vi "plot_id_extractor.vi"(10 "Plot processed data In":T1={"Plot Rep Arrays"=[], "Graph Range Min/Max"={"X"={"Min"=0.0, "Max"=-inf}, "Y"={"Min"=0.0, "Max"=-inf}, "Z"={"Min"=inf, "Max"=-inf}, "Amplitude"={"Min"=0.0, "Max"=0.0}}} caption="Data In") -> (1 "Plot IDs":i32[](array[numeric]), 2 "Plot processed data Out":T1={"Plot Rep Arrays"=[], "Graph Range Min/Max"={"X"={"Min"=0.0, "Max"=-inf}, "Y"={"Min"=0.0, "Max"=-inf}, "Z"={"Min"=inf, "Max"=-inf}, "Amplitude"={"Min"=0.0, "Max"=0.0}}} caption="Data Out")   [LabVIEW 2020, in "3DPC_SurfacePlot.xctl"]
uses:
  <vilib>/Native 3D Graph/xcontrol/3DPC_SurfacePlot.xctl
  <vilib>/Native 3D Graph/xcontrol/Processed Data.ctl
  <vilib>/Native 3D Graph/typedefs/plot_rep_array.ctl
  <vilib>/Native 3D Graph/typedefs/plot_rep.ctl
  <vilib>/Native 3D Graph/typedefs/range_cluster.ctl
  <vilib>/Native 3D Graph/typedefs/min_max.ctl
  <vilib>/Native 3D Graph/typedefs/plot_rep_mesh_data.ctl
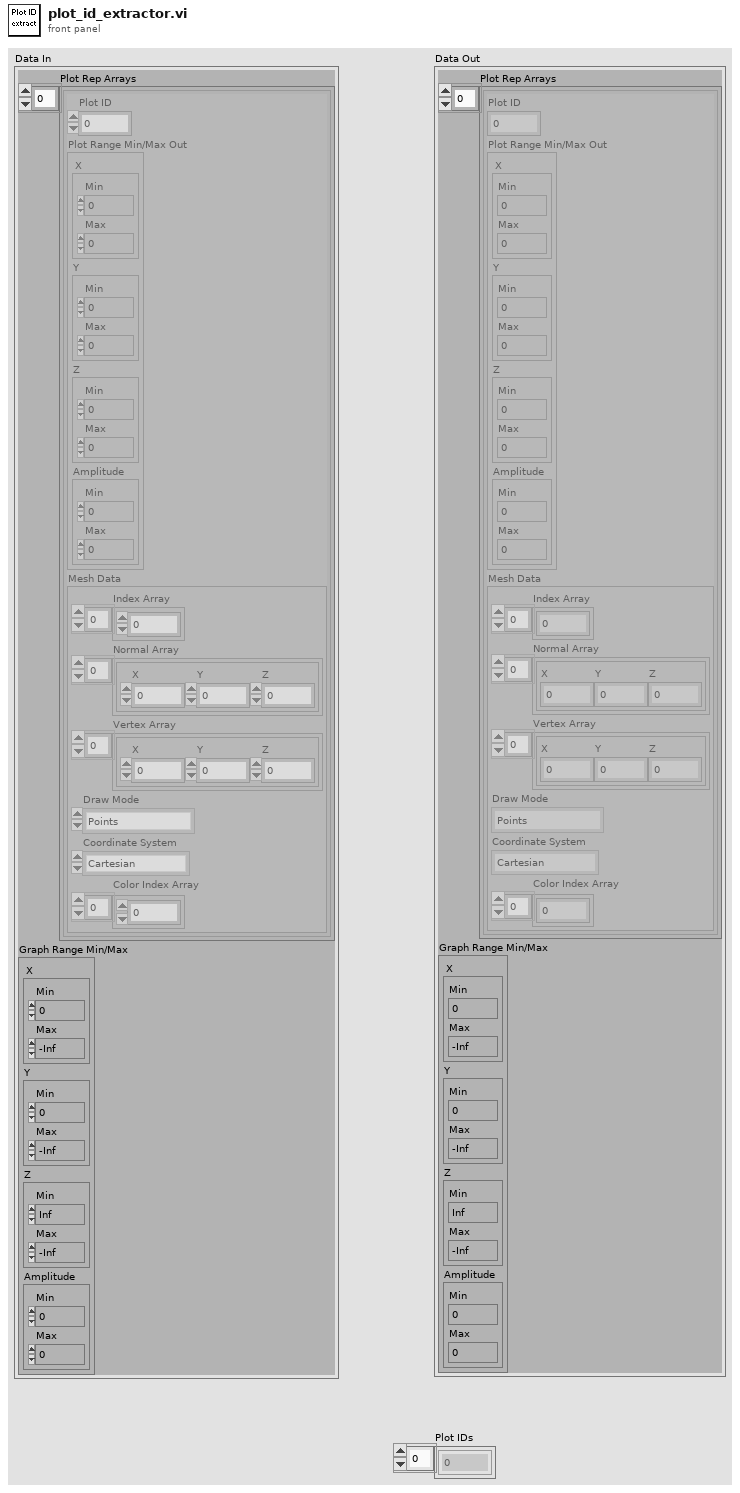
[diagram p1: front panel]
types:
  T1 = typedef "Processed Data.ctl" = cluster{"Plot Rep Arrays":T2, "Graph Range Min/Max":T4}
  T2 = typedef "3DPC_SurfacePlot.xctl/plot_rep_array.ctl" = T3[]
  T3 = typedef "3DPC_SurfacePlot.xctl/plot_rep.ctl" = cluster{"Plot ID":i32, "Plot Range Min/Max Out":T4, "Mesh Data":T6}
  T4 = typedef "3DPC_SurfacePlot.xctl/range_cluster.ctl" = cluster{"X":T5, "Y":T5, "Z":T5, "Amplitude":T5}
  T5 = typedef "3DPC_SurfacePlot.xctl/min_max.ctl" = cluster{"Min":sgl, "Max":sgl}
  T6 = typedef "3DPC_SurfacePlot.xctl/plot_rep_mesh_data.ctl" = cluster{"Index Array":u32[], "Normal Array":cluster{"X":sgl, "Y":sgl, "Z":sgl}[], "Vertex Array":cluster{"X":sgl, "Y":sgl, "Z":sgl}[], "Draw Mode":enum16{"Points", "Lines", "Line Strip", "Line Loop", "Triangles", "Triangle Strip", "Triangle Fan", "Quads", "Quad Strip", "Polygon"}, "Coordinate System":enum16{"Cartesian", "Cylindrical", "Spherical"}, "Color Index Array":i32[]}
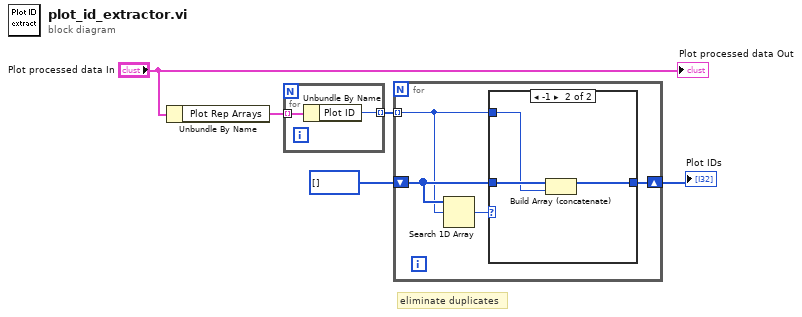
[diagram p0: block diagram]
diagram:
  # "eliminate duplicates"
  n1 = Unbundle By Name("Plot processed data In") -> ("Plot Rep Arrays"=w3:T2)
  n2 = for {
    tunnel: w3 -> [w7] mode=indexing
    tunnel: [w6] -> w2 mode=indexing
    n3 = Unbundle By Name(w7) -> ("Plot ID"=w6:i32)
  }
  n4 = for {
    tunnel: w2 -> [w9] mode=indexing
    shift-right: [w10] -> w4
    shift-left: i32[] [] -> [w11]
    n5 = Search 1D Array(1D array=w11, element=w9) -> (index of element=w8:i32)  [unwired: 1 out]
    n6 = case shown="-1" w8 {
      tunnel: w11 -> [w12 w15]
      tunnel: w9 -> [_ w14]
      tunnel: [w12 w13] -> w10
      frame Default {
      }
      frame -1 {
        n7 = Build Array (concatenate)(w15, w14) -> (w13:i32[])
      }
    }
  }
  "Plot IDs" <- w4
  "Plot processed data Out" <- "Plot processed data In"
